vi "Asynchronous - BC Command Channels - Send Acyclic Messages.vi"(7 "Map (Bc Acyclic Messages Trigger)":T1[](array[typedef]) {"Acyclic Message Trigger Channel Ref" format="%.0x"}, 8 "Error (in)":errorcluster, 11 "Changes?":bool[](array[boolean])) -> (0 "Error (out)":errorcluster)   [LabVIEW 2017, in "Ballard MIL-1553 Engine.lvlib"]
uses:
  Ballard MIL-1553 Engine.lvlib
  Controls/RT Async_Map BC Acyclic Messages Trigger.ctl
  Controls/RT Async_Map_Type.ctl
  <vilib>/NI Veristand/Custom Device API/Custom Device Item Ref.ctl
  <instrlib>/BTI1553Lib/Private/BC/Data/BC Transmit Acyclic Frame.vi
  <instrlib>/BTI1553Lib/BTI1553LV.lvlib
  <vilib>/NI VeriStand/Custom Device Tools/Custom Device Utility Library/Custom Device Utility Library.lvlib
  <vilib>/NI VeriStand/Custom Device API/Custom Device API.lvlib
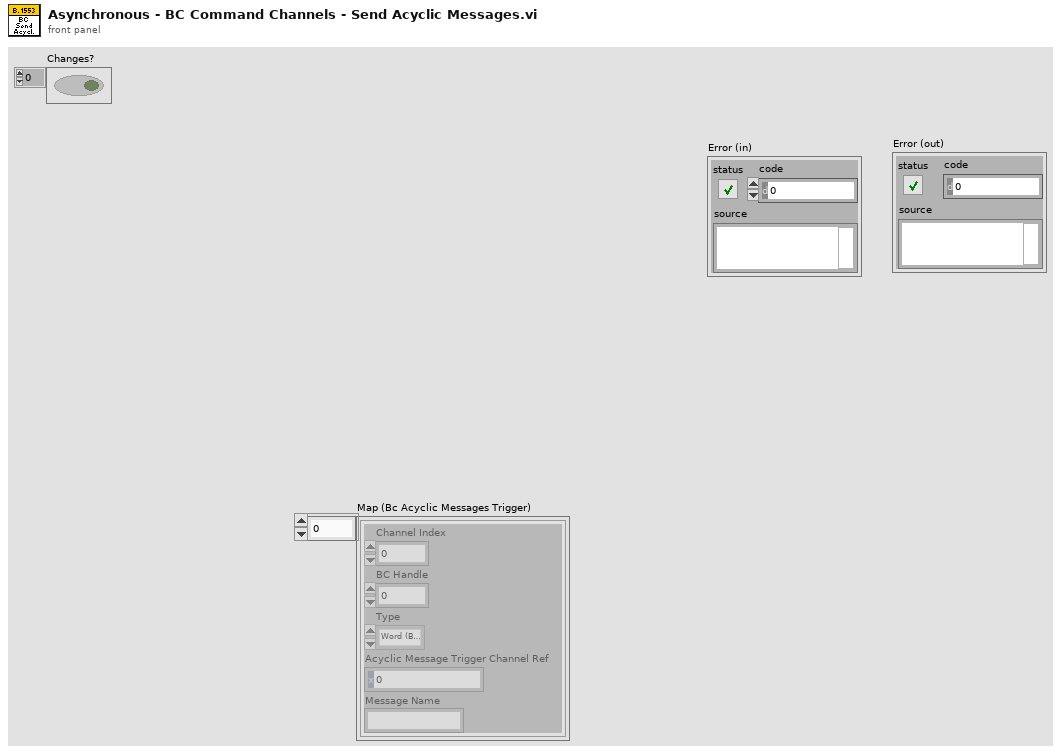
[diagram p1: front panel]
types:
  T1 = typedef "Ballard MIL-1553 Engine.lvlib/RT Async_Map BC Acyclic Messages Trigger.ctl" = cluster{"Channel Index":i32, "BC Handle":u64, "Type":T2, "Acyclic Message Trigger Channel Ref":T3, "Message Name":string}
  T2 = typedef "Ballard MIL-1553 Engine.lvlib/RT Async_Map_Type.ctl" = enum16{"Word (BC to RT)", "Word (MC (Rx))", "Acyclic Message Trigger", "Word (RT to ..)", "Word (RT to RT)", "Word (MC (Tx))", "RT Status", "BC Commands", "RT Commands"}
  T3 = typedef "Custom Device API.lvlib/Custom Device Item Ref.ctl" = u64
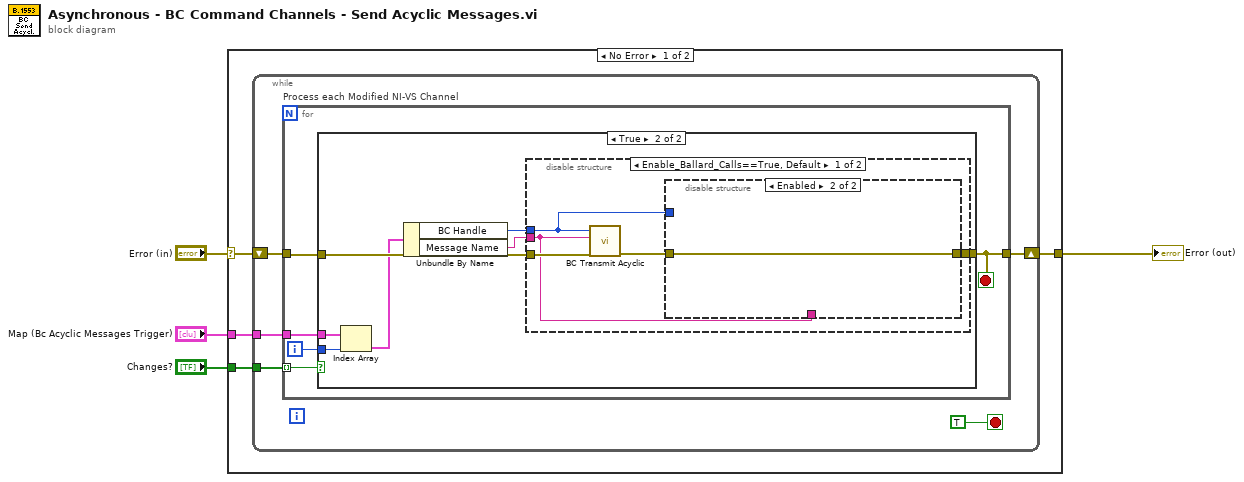
[diagram p0: block diagram]
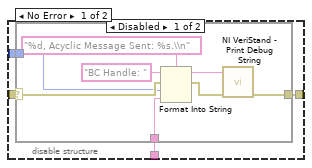
[diagram p3: hidden frame]
diagram:
  n1 = case shown="No Error" "Error (in)" {
    selector: "Error (in)" -> [w5 w47]
    tunnel: "Changes?" -> [w8 _]
    tunnel: [w7 w47] -> w3
    tunnel: "Map (Bc Acyclic Messages Trigger)" -> [w6 _]
    frame No Error {
      n2 = while {
        tunnel: w8 -> [w13]
        tunnel: w6 -> [w10]
        shift-right: [w11] -> w7
        shift-left: w5 -> [w12]
        stop <- TRUE stop-if-true
        n3 = for "Process each Modified NI-VS Channel" {
          tunnel: w13 -> [w14] mode=indexing
          tunnel: w12 -> [w18]
          tunnel: [w16] -> w11
          tunnel: w10 -> [w17]
          i -> [w15]
          stop <- w16 stop-if-true
          n4 = case shown="True" w14 {
            tunnel: w18 -> [w19 w26]
            tunnel: w17 -> [_ w25]
            tunnel: [w19 w24] -> w16
            tunnel: w15 -> [_ w23]
            frame False {
            }
            frame True {
              n5 = Index Array(array=w25, index=w23) -> (element=w22:T1)
              n6 = Unbundle By Name(w22) -> ("BC Handle"=w21:u64, "Message Name"=w20:string)
              n7 = disable-structure shown="Enable_Ballard_Calls==True, Default" {
                disable-tunnel: w26 -> [w31 w46]
                disable-tunnel: [w29 w46] -> w24
                disable-tunnel: w21 -> [w28 _]
                disable-tunnel: w20 -> [w27 _]
                frame condition #0 (active) {
                  n8 = call-poly <instrlib>:"BC Transmit Acyclic.vi"("error in (no error)"=w31, "acyclic frame name"=w27, "bus controller handle in"=w28) -> ("error out"=w30:errorcluster)  [unwired: 7 in, 1 out]
                  n9 = disable-structure shown="Enabled" {
                    disable-tunnel: w30 -> [w35 w45]
                    disable-tunnel: [w34 w45] -> w29
                    disable-tunnel: w28 -> [w33 _]
                    disable-tunnel: w27 -> [w32 _]
                    frame Disabled {
                      n10 = case shown="No Error" w35 {
                        selector: w35 -> [w38 w44]
                        tunnel: [w42 w44] -> w34
                        tunnel: w33 -> [w37 _]
                        tunnel: w32 -> [w36 _]
                        frame No Error {
                          n11 = Format Into String(format string="%d, Acyclic Message Sent: %s.\\n", initial string="BC Handle: ", error in=w38, w37, w36) -> (resulting string=w43:string, error out=w39:errorcluster)
                          n12 = call <vilib>:"NI VeriStand - Print Debug String.vi"("error in (no error)"=w39, "Message"=w43) -> ("error out"=w42:errorcluster)  [unwired: 9 in]
                        }
                        frame Error {
                        }
                      }
                    }
                    frame Enabled {
                    }
                  }
                }
                frame condition #1 {
                }
              }
            }
          }
        }
      }
    }
    frame Error {
    }
  }
  "Error (out)" <- w3
